vi "zad3.vi"() -> ()   [LabVIEW 2017]
panel:
  out "Lampa Uliczna":cluster{"1":bool, "2":bool, "3":bool}
  out "error out":errorcluster
  in  "error in (no error)":errorcluster
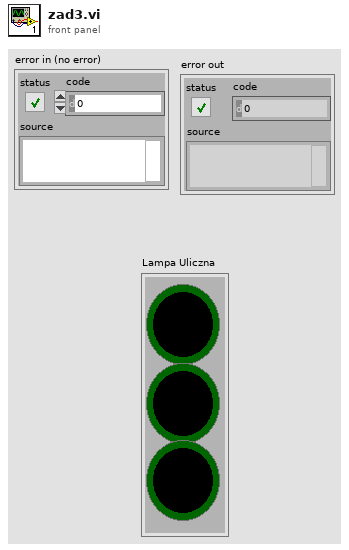
[diagram p1: front panel]
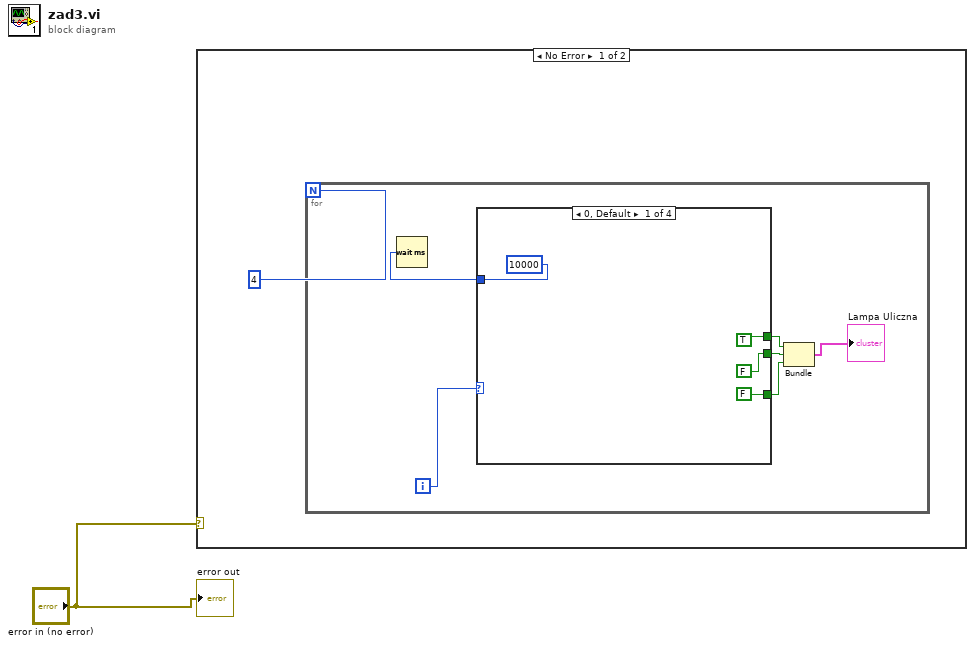
[diagram p0: block diagram]
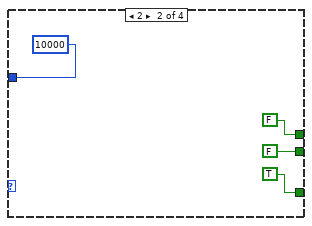
[diagram p2: hidden frame]
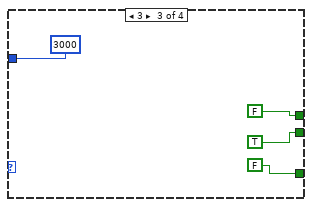
[diagram p3: hidden frame]
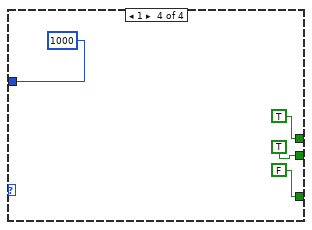
[diagram p4: hidden frame]
diagram:
  n1 = case shown="No Error" "error in (no error)" {
    frame No Error {
      n2 = for {
        N: 4 -> [_]
        i -> [w8]
        n3 = case shown="0, Default" w8 {
          tunnel: [FALSE ("2") FALSE ("2") TRUE ("2") TRUE ("2")] -> w6
          tunnel: [FALSE ("3") TRUE ("3") FALSE ("3") FALSE ("3")] -> w5
          tunnel: [TRUE ("1") FALSE ("1") FALSE ("1") TRUE ("1")] -> w4
          tunnel: [10000 10000 3000 1000] -> w3
          frame 0, Default {
          }
          frame 2 {
          }
          frame 3 {
          }
          frame 1 {
          }
        }
        n4 = Wait (ms)(milliseconds to wait=w3) -> ()  [unwired: 1 out]
        n5 = Bundle("1"=w4, "2"=w6, "3"=w5) -> (→"Lampa Uliczna":cluster{"1":bool, "2":bool, "3":bool})  [unwired: 1 in]
      }
    }
    frame Error {
    }
  }
  "error out" <- "error in (no error)"
